vi "Write Movie Appearances.vi"(8 "error in (no error)":errorcluster, 10 "Movie Appearances":string, 11 "Chevy Chase in":refnum<class "Chevy Chase.lvclass">) -> (0 "error out":errorcluster, 3 "Chevy Chase out":refnum<class "Chevy Chase.lvclass">)   [LabVIEW 2019, in "Chevy Chase.lvclass"]
uses:
  Chevy Chase.lvclass
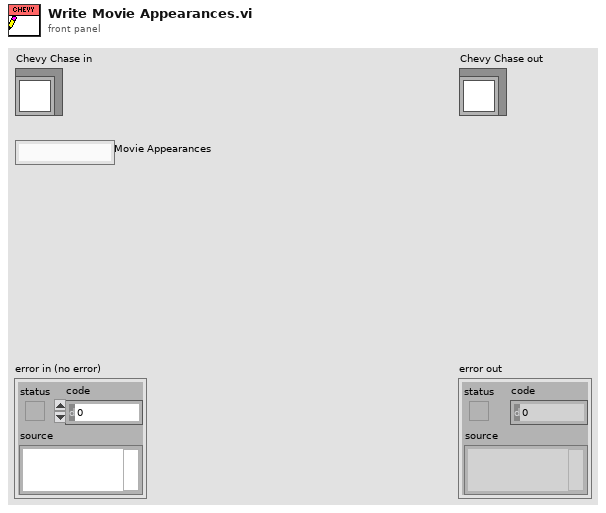
[diagram p1: front panel]
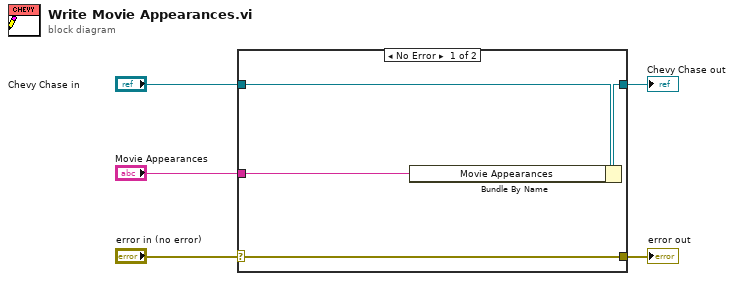
[diagram p0: block diagram]
diagram:
  n1 = case shown="No Error" "error in (no error)" {
    selector: "error in (no error)" -> [w9 w10]
    tunnel: [w9 w10] -> w4
    tunnel: [w7 w11] -> w2
    tunnel: "Chevy Chase in" -> [w8 w11]
    tunnel: "Movie Appearances" -> [w6 _]
    frame No Error {
      n2 = Bundle By Name(cluster=w8, "Movie Appearances"=w6) -> (w7:refnum<class "Chevy Chase.lvclass">)
    }
    frame Error {
    }
  }
  "error out" <- w4
  "Chevy Chase out" <- w2
